vi "Query Resistance.vi"(8 "error in":errorcluster, 11 "2727 in":refnum<class "2727.lvclass">) -> (0 "error out":errorcluster, 2 "Resistance":dbl[](array[numeric]), 3 "2727 out":refnum<class "2727.lvclass">)   [LabVIEW 2019, in "2727.lvlib" / "2727.lvclass"]
uses:
  Library/2727.lvclass
  C:/Users/Public/Documents/Development/builds/Instruments/PRM.lvlibp/Library/PRM.lvclass
  Library/2727.lvclass/2727.ctl
  <instrlib>/ni272xReferenceVIs/ni272xReferenceVIs.llb/ni272x Attribute ID Channel Single.ctl
  builds/Instruments/PRM.lvlibp/Accessors/Read NumChans.vi
  <instrlib>/ni272xReferenceVIs/ni272xReferenceVIs.llb/ni272x Get Attribute Channel Single.vi
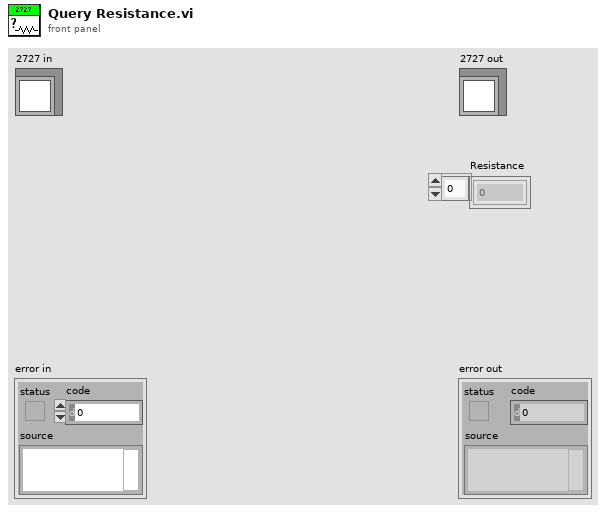
[diagram p1: front panel]
types:
  T1 = typedef "ni272x Attribute ID Channel Single.ctl" = enum16{"Minimum Resistance", "Maximum Resistance", "Resistance"}
  T2 = typedef "ni272x Reference.ctl" = refnum<k20>
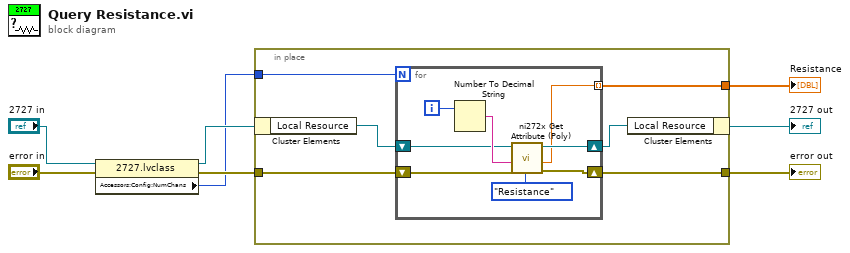
[diagram p0: block diagram]
diagram:
  n1 = property class="2727.lvclass"(reference="2727 in", error in="error in") -> (reference out=w2:refnum<class "2727.lvclass">, error out=w4:errorcluster, "Accessors:Config:NumChans"=w1:i32)
  n2 = in-place {
    in-place-border: w4 -> [w12]
    in-place-border: [w11] -> w6
    in-place-border: [w10] -> w5
    in-place-border: w1 -> [w9]
    n3 = in-place-cluster #1(w2) -> ("Local Resource"=w14:T2)
    n4 = for {
      N: w9 -> [_]
      shift-right: [w19] -> w13
      shift-left: w14 -> [w20]
      shift-right: [w17] -> w11
      shift-left: w12 -> [w16]
      tunnel: [w15] -> w10 mode=indexing
      i -> [w18]
      n5 = Number To Decimal String(number=w18) -> (decimal integer string=w22:string)  [unwired: 1 in]
      n6 = call-poly <instrlib>:"ni272x Get Attribute (Poly).vi"("error in (no error)"=w16, "resistor channel"=w22, "attribute ID channel single"=ni272x_Attribute_ID_Channel_Single."Resistance", "instrument handle"=w20) -> ("error out"=w17:errorcluster, "channel single attribute value"=w15:sgl, "instrument handle out"=w19:T2)  [unwired: 5 in]
    }
    n7 = in-place-cluster #1("Local Resource"=w13) -> (→"2727 out":refnum<class "2727.lvclass">)
  }
  "error out" <- w6
  "Resistance" <- w5
